vi "Pre.vi"(7 "Datum":refnum<class "Datum.lvclass">, 8 "Error In":errorcluster, 10 "Tag In":refnum<class "Variable.lvclass">, 11 "Pre-Mock Render Variable Hook In":refnum<class "Mock Render Variable Hook.lvclass">) -> (0 "Error Out":errorcluster, 2 "Tag Out":refnum<class "Variable.lvclass">, 3 "Pre-Mock Render Variable Hook Out":refnum<class "Mock Render Variable Hook.lvclass">)   [LabVIEW 2018, in "Tests.lvlib" / "Render.lvlib" / "Mock Render Variable Hook.lvclass"]
uses:
  Mock Render Variable Hook.lvclass
  src/Toolkit/Low-Level/Nodes/Variable/Variable.lvclass
  src/Toolkit/Data/Datum/Datum.lvclass
  src/Toolkit/Hooks/Pre-Render Variable/Render Variable.lvclass
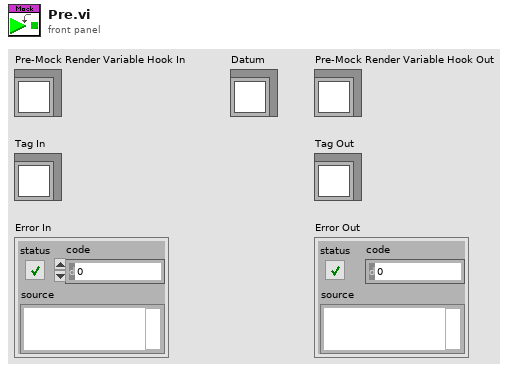
[diagram p1: front panel]
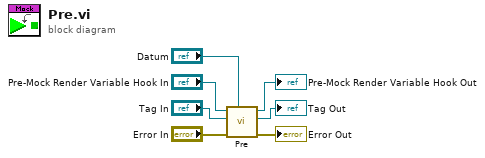
[diagram p0: block diagram]
diagram:
  n1 = call-parent "Pre.vi"("Datum"="Datum", "Error In"="Error In", "Tag In"="Tag In", "Pre-Render Variable In"="Pre-Mock Render Variable Hook In") -> ("Error Out"=→"Error Out":errorcluster, "Tag Out"=→"Tag Out":refnum<class "Variable.lvclass">, "Pre-Render Variable Out"=→"Pre-Mock Render Variable Hook Out":refnum<class "Mock Render Variable Hook.lvclass">)  [unwired: 5 in]
